vi "Do Command.vi"(6 "Actions In":refnum<class "Iteration Actions.lvclass">, 7 "Variables in":refnum<class "Variables.lvclass">, 8 "error in (no error)":errorcluster, 9 "Sequence Time":T1, 10 "VolatusAPI":refnum<class "VolatusAPI.lvclass">, 11 "Stop Seq Command in":refnum<class "Stop Seq Command.lvclass">) -> (0 "error out":errorcluster, 4 "Actions":refnum<class "Iteration Actions.lvclass">, 5 "Variables":refnum<class "Variables.lvclass">)   [LabVIEW 2020, in "VolatusSeq.lvlib" / "Stop Seq Command.lvclass"]
uses:
  Stop Seq Command.lvclass
  Stop Seq Command.lvclass/Stop Seq Command.ctl
  Iteration Actions/Iteration Actions.lvclass
  Variables/Variables.lvclass
  Volatus/VolatusAPI/VolatusAPI.lvclass
  Sequence Time.ctl
  VolatusSeq.lvlib
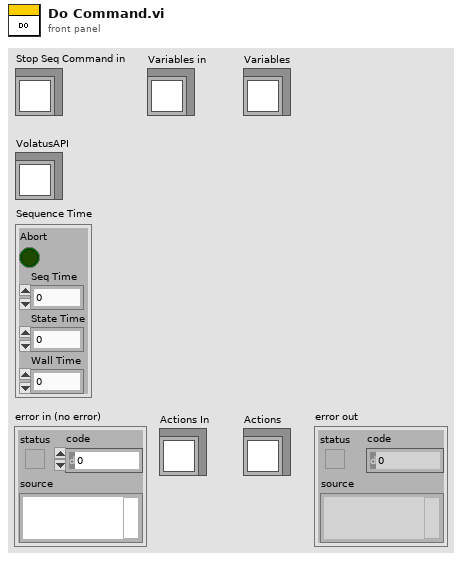
[diagram p1: front panel]
types:
  T1 = typedef "VolatusSeq.lvlib/Sequence Time.ctl" = cluster{"Abort":bool, "Seq Time":dbl, "State Time":dbl, "Wall Time":dbl}
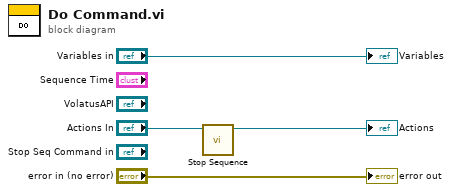
[diagram p0: block diagram]
diagram:
  n1 = call "Stop Sequence.vi"("Iteration Actions in"="Actions In") -> ("Iteration Actions out"=→"Actions":refnum<class "Iteration Actions.lvclass">)  [unwired: 9 in, 1 out]
  "error out" <- "error in (no error)"
  "Variables" <- "Variables in"
